vi "CheckGyroTimeout.vi"(11 "GyroRxLoopData in":T1={"State"=enum."ReadHeader3", "Timestamp"=0, "Timeout"=0, "CRC"=0, "Checksum"=0, "IsLBIT"=FALSE, "ReservedCount"=0, "SBITSample"={"Timestamp"=0, "TxBytes"=0, "RxBytes"=0, "TxFrames"=0, "RxFrames"=0, "BIT0"=0, "BIT1"=0, "BIT2"=0, "BIT3"=0, "BIT4"=0, "BIT5"=0}, "LBITSample"={"Timestamp"=0, "TxBytes"=0, "RxBytes"=0, "TxFrames"=0, "RxFrames"=0, "BIT0"=0, "BIT1"=0, "BIT2"=0, "BIT3"=0, "BIT4"=0, "BIT5"=0, "BIT6"=0, "BIT7"=0}, "Sample"={"Timestamp"=0, "TxBytes"=0, "RxBytes"=0, "TxFrames"=0, "RxFrames"=0, "GyroX"=0, "GyroY"=0, "GyroZ"=0, "Status"=0, "SequenceNumber"=0, "Temperature"=0}, "ErrorSample"={"Timestamp"=0, "TxBytes"=0, "RxBytes"=0, "TxFrames"=0, "RxFrames"=0, "ErrorCode"=enum."None"}}) -> (3 "GyroRxLoopData out":T1={"State"=enum."ReadHeader3", "Timestamp"=0, "Timeout"=0, "CRC"=0, "Checksum"=0, "IsLBIT"=FALSE, "ReservedCount"=0, "SBITSample"={"Timestamp"=0, "TxBytes"=0, "RxBytes"=0, "TxFrames"=0, "RxFrames"=0, "BIT0"=0, "BIT1"=0, "BIT2"=0, "BIT3"=0, "BIT4"=0, "BIT5"=0}, "LBITSample"={"Timestamp"=0, "TxBytes"=0, "RxBytes"=0, "TxFrames"=0, "RxFrames"=0, "BIT0"=0, "BIT1"=0, "BIT2"=0, "BIT3"=0, "BIT4"=0, "BIT5"=0, "BIT6"=0, "BIT7"=0}, "Sample"={"Timestamp"=0, "TxBytes"=0, "RxBytes"=0, "TxFrames"=0, "RxFrames"=0, "GyroX"=0, "GyroY"=0, "GyroZ"=0, "Status"=0, "SequenceNumber"=0, "Temperature"=0}, "ErrorSample"={"Timestamp"=0, "TxBytes"=0, "RxBytes"=0, "TxFrames"=0, "RxFrames"=0, "ErrorCode"=enum."None"}})   [LabVIEW 2018]
uses:
  GyroRxLoopData.ctl
  GyroRxLoopStates.ctl
  GyroSBITSample.ctl
  GyroLBITSample.ctl
  GyroSample.ctl
  GyroErrorSample.ctl
  GyroErrorCodes.ctl
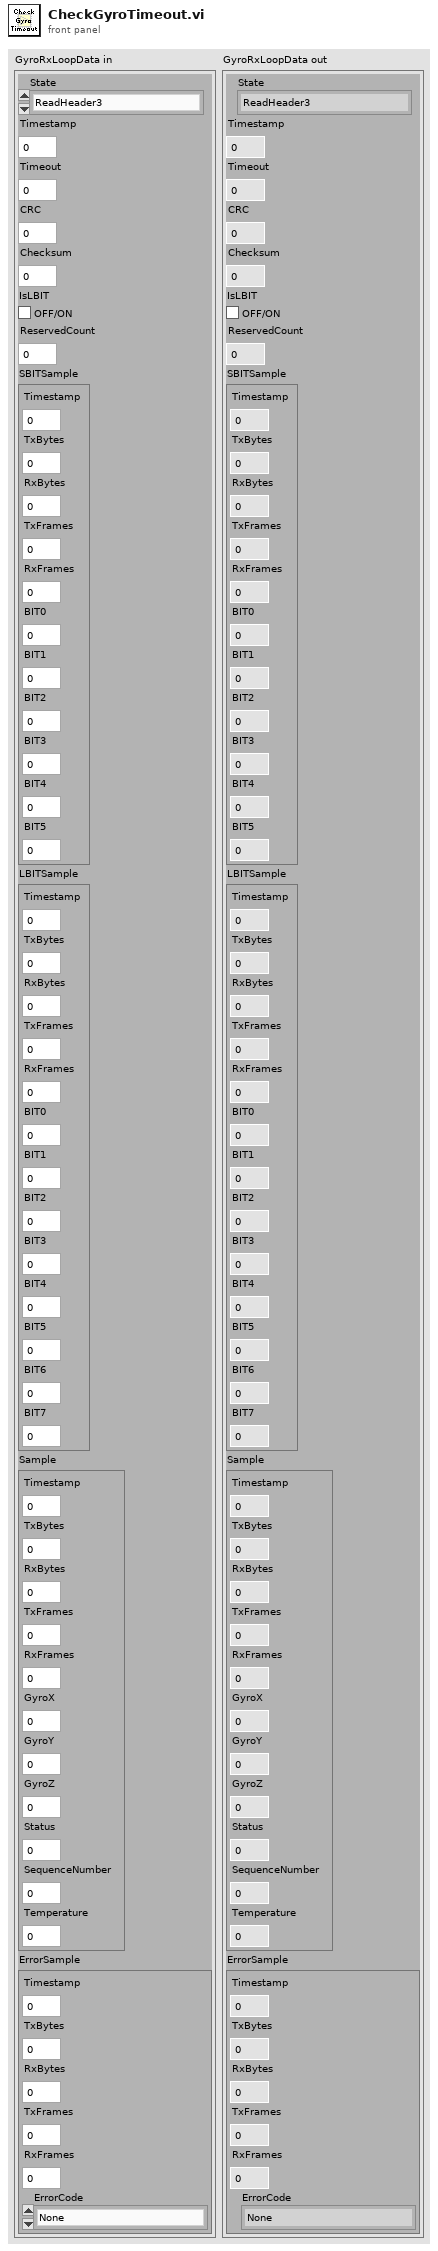
[diagram p1: front panel]
types:
  T1 = typedef "GyroRxLoopData.ctl" = cluster{"State":T2, "Timestamp":u64, "Timeout":i32, "CRC":u32, "Checksum":u8, "IsLBIT":bool, "ReservedCount":u8, "SBITSample":T3, "LBITSample":T4, "Sample":T5, "ErrorSample":T6}
  T2 = typedef "GyroRxLoopStates.ctl" = enum16{"WaitForSilence", "ReadHeader3", "IgnoreASCIIResponse", "ReadNormalHeader2", "ReadNormalHeader1", "ReadBITHeader0", "ReadBIT0", "ReadBIT1", "ReadBIT2", "ReadBIT3", "ReadBIT4", "ReadBIT5", "ReadBIT6", "ReadBIT7", "ReadChecksum", "PrepareSBIT", "MoveSBIT", "PrepareLBIT", "MoveLBIT", "ReadSampleHeader0", "ReadSampleX3", "ReadSampleX2", "ReadSampleX1", "ReadSampleX0", "ReadSampleY3", "ReadSampleY2", "ReadSampleY1", "ReadSampleY0", "ReadSampleZ3", "ReadSampleZ2", "ReadSampleZ1", "ReadSampleZ0", "ReadSampleReserved", "ReadSampleStatus", "ReadSampleSequenceNumber", "ReadSampleTemperature1", "ReadSampleTemperature0", "ReadSampleCRC3", "ReadSampleCRC2", "ReadSampleCRC1", "ReadSampleCRC0", "VerifyCRC", "PrepareSample", "MoveSample", "ResponseHeaderError", "ResponseCRCError", "ResponseTimeoutError", "ResponseChecksumError", "PrepareErrorCode", "MoveErrorCode", "ClearCRC", "WaitForCRCCleared"}
  T3 = typedef "GyroSBITSample.ctl" = cluster{"Timestamp":u64, "TxBytes":u64, "RxBytes":u64, "TxFrames":u64, "RxFrames":u64, "BIT0":u8, "BIT1":u8, "BIT2":u8, "BIT3":u8, "BIT4":u8, "BIT5":u8}
  T4 = typedef "GyroLBITSample.ctl" = cluster{"Timestamp":u64, "TxBytes":u64, "RxBytes":u64, "TxFrames":u64, "RxFrames":u64, "BIT0":u8, "BIT1":u8, "BIT2":u8, "BIT3":u8, "BIT4":u8, "BIT5":u8, "BIT6":u8, "BIT7":u8}
  T5 = typedef "GyroSample.ctl" = cluster{"Timestamp":u64, "TxBytes":u64, "RxBytes":u64, "TxFrames":u64, "RxFrames":u64, "GyroX":u32, "GyroY":u32, "GyroZ":u32, "Status":u8, "SequenceNumber":u8, "Temperature":i16}
  T6 = typedef "GyroErrorSample.ctl" = cluster{"Timestamp":u64, "TxBytes":u64, "RxBytes":u64, "TxFrames":u64, "RxFrames":u64, "ErrorCode":T7}
  T7 = typedef "GyroErrorCodes.ctl" = enum8{"None", "ResponseHeaderError", "ResponseCRCError", "ResponseTimeoutError", "ResponseChecksumError"}
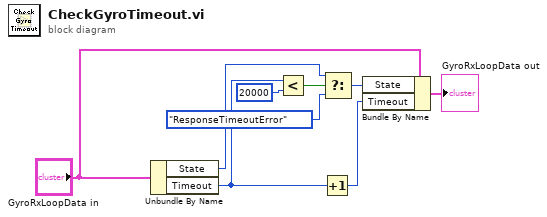
[diagram p0: block diagram]
diagram:
  n1 = Unbundle By Name("GyroRxLoopData in") -> ("State"=w9:T2, "Timeout"=w8:i32)
  n2 = Less?(x=w8, y=20000) -> (x < y?=w7:bool)
  n3 = Increment(x=w8) -> (x+1=w2:i32)
  n4 = Select(t=w9, s=w7, f=GyroRxLoopStates."ResponseTimeoutError" ("GyroRxLoopStates")) -> (s? t:f=w3:T2)
  n5 = Bundle By Name(cluster="GyroRxLoopData in", "State"=w3, "Timeout"=w2) -> (→"GyroRxLoopData out":T1)
